vi "Write Flat Configuration.vi"(8 "error in (no error)":errorcluster, 10 "Configuration":variant, 11 "CIFTemplateNode in":refnum<class "CIFCorePlugin.lvclass">) -> (0 "error out":errorcluster, 3 "CIFTemplateNode out":refnum<class "CIFCorePlugin.lvclass">)   [LabVIEW 2021, in "CIFCorePlugin.lvclass"]
uses:
  CIFCorePlugin.lvclass
  CIFUtilities/CIFLogs/Typedef/Plugin State Commands.ctl
  CIFCorePlugin.lvclass/CIFCorePlugin.ctl
  CIFUtilities/CIFOutOfBand/CIFOutOfBand.lvclass/CIFOutOfBand.ctl
  Read Plugin Name.vi
  Read Version.vi
  CIFUtilities/CIFOutOfBand/Accessors/Write Local OOB Data.vi
  CIFUtilities/CIFOutOfBand/Accessors/Read Local OOB Data.vi
  OOB/OOB_Rx/CIFCoreOOB_Rx.lvclass
  D:/dev/CIF-LVCore/src/CIFUtilities/CIFOutOfBand/CIFOutOfBand.lvclass
  <vilib>/addons/_JKI.lib/Serialization/JSON/JKI JSON Serialization.lvlib
  CIFUtilities/CIFLogs/CIFLogs.lvlib
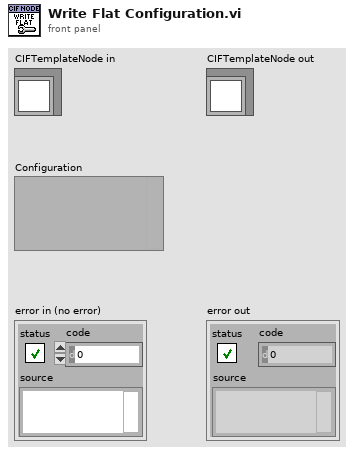
[diagram p1: front panel]
types:
  T1 = typedef "CIFLogs.lvlib/Plugin State Commands.ctl" = enum16{"Create", "Configure", "Run", "Pause", "Destroy", "Connect", "Force"}
  T2 = typedef "CIFCoreCommon.lvlib/Version.ctl" = cluster{"Major":i32, "Minor":i32, "Fix":i32, "Build":i32}
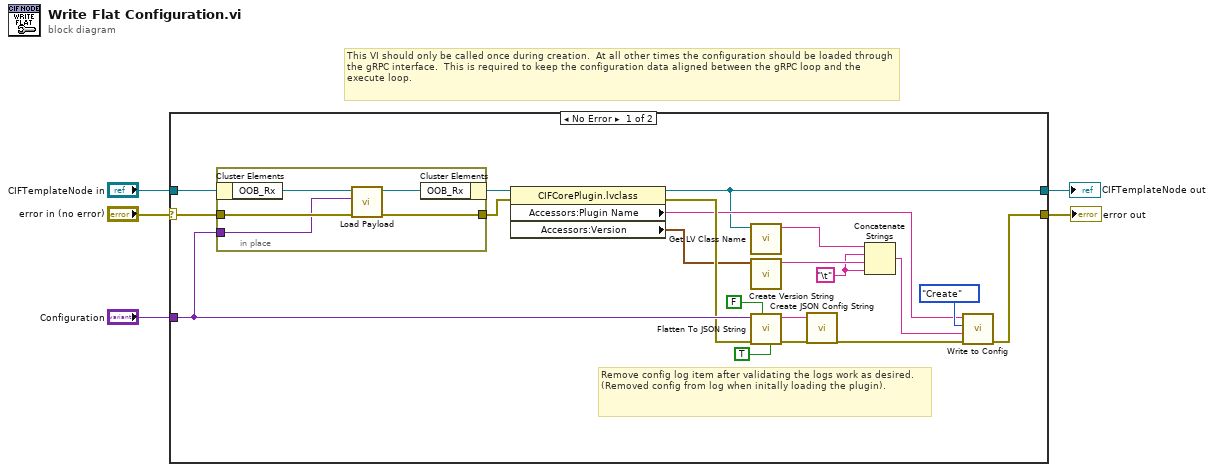
[diagram p0: block diagram]
diagram:
  # "This VI should only be called once during creation.  At all other times the configuration should be loaded through the gRPC interface.  This is required to keep the configuration data aligned between the gRPC loop and the execute loop."
  n1 = case shown="No Error" "error in (no error)" {
    selector: "error in (no error)" -> [w23 w30]
    tunnel: [w19 w30] -> w4
    tunnel: [w9 w31] -> w2
    tunnel: "CIFTemplateNode in" -> [w24 w31]
    tunnel: "Configuration" -> [w22 _]
    frame No Error {
      w6 = "\t"
      # "Remove config log item after validating the logs work as desired.  (Removed config from log when initally loading the plugin)."
      n2 = in-place {
        in-place-border: w23 -> [w27]
        in-place-border: [w26] -> w15
        in-place-border: w22 -> [w25]
        n3 = in-place-cluster #1(w24) -> ("OOB_Rx"=w29:refnum<class "CIFCoreOOB_Rx.lvclass">)
        n4 = call "Load Payload.vi"("error in (no error)"=w27, "Configuration Payload"=w25, "CoreOOB_Rx in"=w29) -> ("error out"=w26:errorcluster, "CoreOOB_Rx out"=w28:refnum<class "CIFCoreOOB_Rx.lvclass">)  [unwired: 7 in]
        n5 = in-place-cluster #1("OOB_Rx"=w28) -> (w16:refnum<class "CIFCorePlugin.lvclass">)
      }
      n6 = property class="CIFCorePlugin.lvclass"(reference=w16, error in=w15) -> (reference out=w9:refnum<class "CIFCorePlugin.lvclass">, error out=w14:errorcluster, "Accessors:Plugin Name"=w13:string, "Accessors:Version"=w8:T2)
      n7 = call <vilib>:"Get LV Class Name.vi"("object"=w9) -> ("class name"=w7:string)  [unwired: 9 in, 1 out]
      n8 = call "Create Version String.vi"("Version"=w8) -> ("Version string"=w12:string)  [unwired: 9 in, 1 out]
      n9 = call <vilib>:"Flatten To JSON String.vi"("Enums As String (F)"=TRUE, "Multiline (T)"=FALSE, "error in (no error)"=w14, "Variant"=w22) -> ("error out"=w18:errorcluster, "JSON String"=w10:string)  [unwired: 6 in]
      n10 = call "Create JSON Config String.vi"("JSON Config"=w10) -> ()  [unwired: 4 in, 1 out]
      n11 = Concatenate Strings(w7, w6, w12, w6) -> (w11:string)
      n12 = call "Write to Config.vi"("error in (no error)"=w18, "Additional Data"=w11, "Command"=Plugin_State_Commands."Create", "Plugin Name"=w13) -> ("error out"=w19:errorcluster)  [unwired: 7 in]
    }
    frame Error {
    }
  }
  "error out" <- w4
  "CIFTemplateNode out" <- w2
